vi "LUT_DrawPlayfield4.vi"() -> (0 "Init Data Out":fxp<+,3,3>[](array[numeric]))   [LabVIEW 2018]
panel:
  in  "DefaultValues":u8[][](array[ring])=[[0, 0, 0, 0, 5, 0, 0, 0, 0, 0], [0, 0, 0, 5, 5, 5, 0, 0, 0, 0], [0, 0, 0, 1, 1, 1, 0, 0, 0, 0], [0, 0, 0, 1, 4, 0, 0, 0, 0, 0], [0, 0, 0, 0, 4, 0, 0, 0, 0, 0], [0, 0, 0, 0, 4, 6, 6, 0, 0, 0], [0, 0, 0, 0, 4, 6, 6, 0, 0, 0], [0, 0, 0, 0, 1, 1, 0, 0, 0, 0], [0, 0, 0, 0, 0, 1, 1, 0, 0, 0], [0, 0, 0, 0, 0, 3, 3, 0, 0, 0], [0, 0, 0, 0, 0, 3, 0, 0, 0, 0], [0, 0, 0, 0, 5, 3, 0, 0, 0, 0], [0, 0, 0, 0, 5, 5, 0, 0, 0, 0], [0, 0, 0, 0, 5, 0, 0, 0, 0, 0], [0, 0, 0, 3, 1, 0, 0, 0, 0, 0], [0, 0, 0, 3, 1, 0, 0, 0, 0, 0], [0, 0, 3, 3, 1, 1, 0, 0, 0, 0], [2, 0, 0, 4, 4, 4, 4, 0, 0, 4], [2, 2, 0, 6, 6, 0, 2, 2, 0, 4], [0, 2, 0, 0, 0, 0, 2, 1, 1, 4]]
  out "size(s)":i32
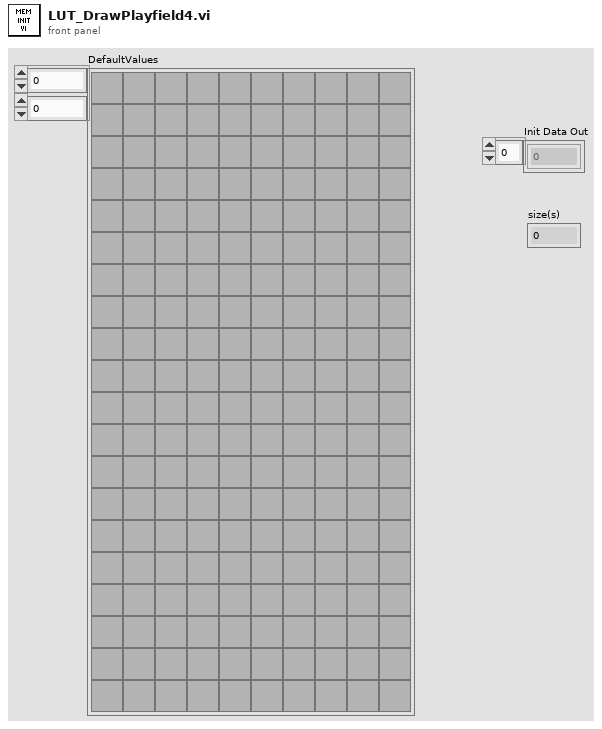
[diagram p1: front panel]
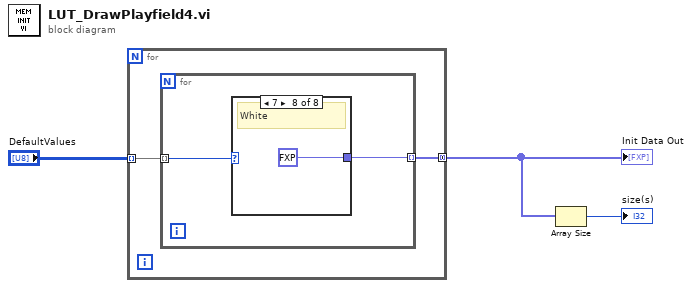
[diagram p0: block diagram]
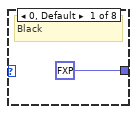
[diagram p2: hidden frame]
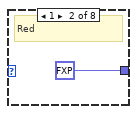
[diagram p3: hidden frame]
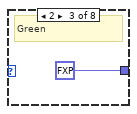
[diagram p4: hidden frame]
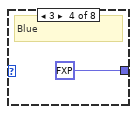
[diagram p5: hidden frame]
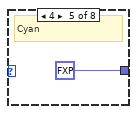
[diagram p6: hidden frame]
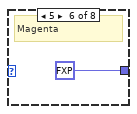
[diagram p7: hidden frame]
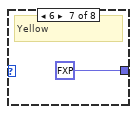
[diagram p8: hidden frame]
diagram:
  n1 = for {
    tunnel: "DefaultValues" -> [w5] mode=indexing
    tunnel: [w4] -> w2 mode=concatenating
    n2 = for {
      tunnel: w5 -> [w7] mode=indexing
      tunnel: [w6] -> w4 mode=indexing
      n3 = case shown="7" w7 {
        tunnel: [fxp<+,1,1> 0.0 fxp<+,1,1> 1.0 fxp<+,1,2> 2.0 fxp<+,1,3> 4.0 fxp<+,2,3> 6.0 fxp<+,3,3> 5.0 fxp<+,2,2> 3.0 fxp<+,3,3> 7.0] -> w6
        frame 0, Default {
          # "Black"
        }
        frame 1 {
          # "Red"
        }
        frame 2 {
          # "Green"
        }
        frame 3 {
          # "Blue"
        }
        frame 4 {
          # "Cyan"
        }
        frame 5 {
          # "Magenta"
        }
        frame 6 {
          # "Yellow"
        }
        frame 7 {
          # "White"
        }
      }
    }
  }
  "Init Data Out" <- w2
  n4 = Array Size(array=w2) -> (size(s)=→"size(s)":i32)
